vi "Sub Navigation.vi"() -> ()   [LabVIEW 2020]
uses:
  command.ctl
  <vilib>/regexp/Match Regular Expression.xnode
panel:
  out "Answer":i32
  in  "Input":string="forward 1\ndown 6\ndown 6\nforward 2\nforward 2\ndown 2\ndown 1\ndown 5\ndown 7\ndown 3\nforward 1\nforward 6\nup 2\nforward 2\nforward 7\nforward 4\ndown 2\nforward 6\nforward 6\ndown 3\nup 7\ndown 6\nforward 2\nup 5\ndown 7\nforward 8\ndown 8\nforward 8\ndown 5\ndown 5\ndown 8\nforward 9\ndown 7\nforward 9\nforward 9\nforward 8\ndown 6\ndown 9\ndown 1\nforward 8\ndown 6\ndown 7\nup 3\nforward 5\ndown 1\ndown 7\nup 8\nforward 6\ndown 2\ndown 9\ndown 9\nforward 1\ndown 2\ndown 9\nforward 1\nforward 3\ndown 6\nup 7\ndown 7\nforward 3\ndown 4\ndown 3\nup 7\nup 7\nforward 2\ndown 7\nforward 2\ndown 3\nup 7\ndown 7\nforward 6\ndown 2\ndown 7\nforward 5\ndown 9\ndown 2\nup 7\ndown 1\nforward 5\ndown 5\nforward 9\ndown 6\ndown 3\ndown 7\ndown 8\ndown 3\nup 4\ndown 6\nforward 6\nup 7\nup 2\nforward 3\nup 1\ndown 5\nforward 9\nup 3\nforward 8\nup 4\ndown 7\ndown 8\ndown 3\ndown 7\nforward 5\nup 6\ndown 4\ndown 8\ndown 8\nforward 7\ndown 5\nforward 3\nforward 1\ndown 1\nforward 1\nup 1\nforward 4\nforward 9\nup 8\ndown 7\ndown 9\ndown 1\ndown 2\ndown 1\ndown 4\nforward 4\nforward 8\nforward 6\nforward 1\nforward 6\nforward 9\ndown 1\nup 9\ndown 9\nforward 2\ndown 6\ndown 8\ndown 6\nup 7\nforward 2\nup 2\nforward 5\ndown 2\nup 2\nup 9\nforward 7\ndown 6\nforward 3\ndown 5\nup 4\ndown 1\ndown 5\ndown 6\nup 7\ndown 3\ndown 9\nup 8\ndown 2\nup 8\ndown 1\ndown 2\ndown 4\nforward 6\nup 7\nup 3\nforward 8\ndown 9\ndown 8\nforward 3\nup 5\nforward 1\ndown 5\nup 2\ndown 5\nup 4\ndown 6\nforward 9\ndown 1\ndown 1\nforward 1\ndown 2\nforward 9\nup 5\ndown 7\nforward 7\ndown 9\ndown 5\ndown 3\nforward 4\ndown 2\nforward 7\nforward 3\nup 4\ndown 9\nforward 9\nforward 3\nforward 1\nforward 6\ndown 1\ndown 5\ndown 3\nforward 9\ndown 2\nforward 9\nup 7\nforward 7\nforward 7\nforward 8\nforward 6\nforward 5\ndown 7\nup 4\nforward 7\nup 2\nforward 6\ndown 2\ndown 9\ndown 3\nforward 5\ndown 3\ndown 9\nforward 2\nup 4\nforward 7\nforward 3\nforward 8\ndown 4\nforward 4\ndown 3\nup 7\nup 1\nup 4\ndown 3\ndown 5\ndown 3\ndown 7\ndown 3\ndown 7\ndown 5\ndown 1\nforward 5\nforward 6\ndown 1\nforward 9\ndown 4\nup 1\nforward 5\nup 6\ndown 4\nup 7\ndown 4\ndown 9\nforward 7\nup 8\nforward 3\nforward 5\ndown 9\ndown 1\ndown 7\nforward 9\ndown 9\ndown 5\nforward 6\nforward 4\nforward 3\ndown 1\ndown 2\nup 4\nup 7\ndown 8\nforward 4\nforward 1\nforward 8\ndown 8\ndown 8\nforward 1\nforward 5\nup 8\nforward 2\ndown 6\nforward 6\ndown 6\nforward 7\ndown 9\ndown 4\nup 4\nup 5\ndown 7\nforward 4\ndown 7\ndown 5\nforward 7\ndown 3\ndown 2\nforward 5\nforward 1\ndown 5\ndown 4\ndown 8\nup 8\nforward 3\ndown 7\ndown 8\ndown 5\nforward 1\ndown 6\nforward 8\nforward 2\nforward 3\ndown 4\nup 3\ndown 4\nforward 3\nforward 9\nup 5\nup 9\ndown 3\nup 4\nforward 4\ndown 9\nforward 8\ndown 2\ndown 2\nforward 9\ndown 5\ndown 2\nup 1\nforward 6\nforward 4\nup 5\nup 3\nup 8\ndown 7\nforward 5\nup 7\nforward 9\ndown 6\ndown 7\nforward 4\ndown 9\nup 2\nforward 8\ndown 1\nforward 6\nforward 1\nforward 4\ndown 9\ndown 6\nup 1\nforward 1\ndown 5\nup 1\nforward 3\ndown 1\ndown 4\nforward 3\ndown 4\nup 9\ndown 6\nup 6\nforward 1\nforward 8\nup 1\ndown 7\nup 8\nup 3\nup 7\ndown 9\nforward 8\ndown 3\nup 2\nforward 3\nup 4\nup 3\ndown 5\nforward 3\nforward 2\ndown 3\nforward 5\nup 4\ndown 9\ndown 8\ndown 3\ndown 5\ndown 7\nforward 2\nforward 8\nup 9\nforward 9\ndown 4\ndown 8\nforward 5\ndown 2\nup 4\ndown 7\nforward 6\nup 9\nforward 6\ndown 9\ndown 5\nforward 9\ndown 5\ndown 3\nup 6\nup 6\ndown 7\nup 1\nforward 7\nforward 4\ndown 5\nforward 8\ndown 5\ndown 8\nforward 4\nforward 8\nforward 1\ndown 7\nforward 4\ndown 6\ndown 4\nup 8\ndown 4\nup 5\nup 7\nup 2\ndown 5\ndown 9\nforward 6\ndown 7\ndown 9\ndown 3\nup 4\ndown 8\nforward 3\nforward 5\nforward 8\ndown 9\nforward 9\ndown 1\nup 1\ndown 9\nforward 3\nup 9\nforward 5\nforward 2\ndown 1\ndown 5\ndown 6\nforward 5\nforward 4\nup 5\nforward 5\nup 4\nup 9\nup 4\nforward 8\ndown 7\ndown 6\ndown 9\ndown 3\ndown 2\ndown 6\nup 6\nforward 6\nup 3\ndown 3\nforward 3\ndown 2\ndown 9\ndown 3\nforward 1\nforward 8\ndown 2\ndown 9\ndown 6\nup 3\ndown 6\nforward 1\nforward 1\nforward 2\ndown 9\ndown 8\nforward 9\ndown 2\nup 3\nforward 2\nup 5\nup 8\ndown 4\nup 3\nforward 3\nforward 5\nforward 1\ndown 5\nup 4\nforward 4\ndown 7\nforward 8\nup 7\nforward 5\ndown 2\nforward 4\nforward 6\ndown 7\ndown 9\nforward 2\nforward 2\ndown 4\ndown 5\nup 5\nforward 5\nforward 2\ndown 8\nforward 6\ndown 1\ndown 6\nforward 1\ndown 8\nup 6\ndown 8\nforward 4\ndown 4\ndown 4\nforward 3\nup 8\ndown 1\nforward 7\ndown 5\nforward 1\ndown 9\ndown 9\ndown 5\nforward 1\ndown 4\nup 6\nforward 4\nforward 5\nforward 1\ndown 4\ndown 2\ndown 5\nforward 6\nforward 1\nforward 6\ndown 2\ndown 6\nforward 3\ndown 9\nup 6\nforward 2\nup 7\nforward 8\ndown 7\nup 1\nforward 1\ndown 8\nforward 8\ndown 9\nforward 4\ndown 4\ndown 5\ndown 8\nup 3\nforward 1\nforward 9\ndown 9\nup 2\ndown 1\ndown 8\ndown 6\nforward 3\ndown 8\ndown 3\nforward 5\nforward 2\nforward 5\nforward 5\nforward 2\nforward 4\ndown 9\ndown 3\nforward 7\nforward 3\nup 3\nup 1\nforward 2\ndown 5\nforward 3\nup 3\nforward 2\nforward 9\nforward 5\ndown 3\nforward 9\nup 2\nforward 7\nup 3\ndown 8\nforward 7\nup 5\nforward 3\nforward 4\nup 5\ndown 6\nup 2\nforward 8\nup 3\ndown 5\ndown 4\nforward 9\nup 2\ndown 5\nforward 4\nup 7\ndown 9\nup 8\ndown 4\nup 5\nforward 4\ndown 8\nforward 3\ndown 5\ndown 5\ndown 8\nup 9\nforward 3\nforward 9\ndown 2\nforward 4\ndown 1\nup 3\ndown 9\nup 6\ndown 1\ndown 1\ndown 5\ndown 1\ndown 7\nforward 4\ndown 4\ndown 9\nup 1\nup 7\nup 2\ndown 8\nup 5\ndown 6\nforward 6\nforward 6\ndown 4\nforward 9\nforward 4\nforward 9\nforward 4\nup 5\nforward 9\nup 7\nup 1\nforward 5\nforward 9\ndown 7\nforward 7\nforward 6\ndown 5\nforward 9\nup 9\ndown 4\ndown 9\ndown 2\nforward 3\ndown 3\ndown 3\nforward 9\ndown 8\ndown 4\ndown 8\ndown 6\ndown 6\ndown 9\nup 5\ndown 3\ndown 4\nup 6\nup 2\nforward 1\nup 9\nup 9\nforward 9\nforward 7\ndown 3\nforward 2\nup 5\ndown 2\nforward 2\nforward 8\ndown 8\nforward 4\nforward 2\nup 3\nup 8\ndown 5\nforward 5\nforward 8\ndown 1\ndown 8\nforward 3\nforward 9\ndown 7\nforward 5\nforward 8\nforward 1\nup 6\nforward 9\nup 5\nforward 8\nforward 3\ndown 2\nup 9\nup 7\nforward 5\ndown 8\ndown 3\nforward 8\ndown 3\ndown 9\ndown 9\nforward 7\ndown 9\nforward 5\nforward 1\nforward 5\ndown 2\ndown 7\nforward 4\ndown 4\nup 8\ndown 2\nup 1\ndown 1\nup 5\nup 6\ndown 5\nup 9\nup 6\ndown 6\ndown 4\ndown 3\nforward 9\nforward 2\nforward 2\nup 6\nforward 9\ndown 3\nforward 4\nforward 6\nforward 8\nforward 2\nforward 8\nforward 4\ndown 1\nforward 3\nup 1\nup 9\nforward 9\nup 6\nup 5\nforward 2\ndown 6\nup 8\nup 9\nforward 3\nforward 9\ndown 7\ndown 6\nforward 2\ndown 7\nforward 4\ndown 5\ndown 2\ndown 6\ndown 2\ndown 5\ndown 3\nforward 3\ndown 7\ndown 6\ndown 5\nup 2\nforward 4\nup 9\nforward 2\nforward 4\ndown 5\nup 9\nup 2\nforward 9\nforward 6\ndown 6\ndown 3\ndown 5\ndown 1\nup 4\nup 1\ndown 4\ndown 1\nforward 5\nforward 3\ndown 7\ndown 9\nforward 2\ndown 3\nup 7\ndown 2\ndown 6\nforward 3\nforward 3\ndown 3\nup 1\nforward 6\nforward 3\ndown 6\ndown 2\nup 4\nup 3\ndown 5\ndown 9\ndown 3\nforward 7\nforward 2\nforward 9\ndown 6\nforward 4\nup 9\nforward 1\ndown 4\ndown 6\ndown 2\nforward 3\ndown 2\nup 8\nforward 1\nforward 9\ndown 9\nup 7\nforward 6\nup 8\ndown 9\ndown 4\nforward 8\ndown 6\ndown 1\ndown 9\ndown 1\nup 7\nforward 9\nup 3\nforward 7\nup 7\ndown 2\nforward 1\ndown 4\ndown 7\nforward 7\nforward 9\ndown 6\ndown 5\ndown 8\ndown 9\nup 3\ndown 7\nup 3\ndown 1\nforward 1\nforward 6\nforward 2\ndown 6\nforward 9\nforward 1\nup 2\nforward 1\nforward 3\nforward 4\nforward 7\nforward 4\ndown 3\nup 8\nforward 9\ndown 7\nforward 6\nforward 3\ndown 6\nforward 4\nup 1\nforward 3\ndown 3\nforward 9\nforward 2\nforward 1\nforward 4\nup 6\nforward 3\ndown 6\ndown 8\nup 4\nforward 8\nforward 4\ndown 8\nup 4\nup 3\nforward 9\nforward 3\ndown 5\nforward 7\nforward 1\nup 8\nup 4\ndown 1\ndown 3\ndown 9\ndown 7\nup 5\nforward 6\ndown 1\nforward 3\ndown 2\ndown 2\ndown 6\nforward 2\ndown 5\nforward 2\nforward 1\nup 9\ndown 1\nforward 3\ndown 3\nforward 6\ndown 1\nforward 5\nforward 7\ndown 6\nforward 7\ndown 4\nup 7\nforward 1\ndown 7\ndown 8\ndown 9\ndown 6\ndown 1\nforward 6\ndown 7\nforward 2\ndown 2\nup 1\nup 2\ndown 3\ndown 4\nup 2\nforward 3\ndown 5\ndown 4\ndown 9\ndown 6\ndown 9\ndown 7\ndown 2\nforward 7\nforward 3\nup 3\ndown 1\ndown 5\ndown 1\ndown 3\ndown 3\nforward 9\ndown 1\ndown 7\nup 4\ndown 1\ndown 6\nup 9\ndown 9\nforward 6\ndown 9\nforward 3\nforward 8\nup 1\nforward 3\ndown 8\nforward 2\ndown 6\ndown 1\nup 7\ndown 1\nforward 3\ndown 2\nforward 1\nup 8\nforward 8\nforward 7\ndown 9\nforward 3"
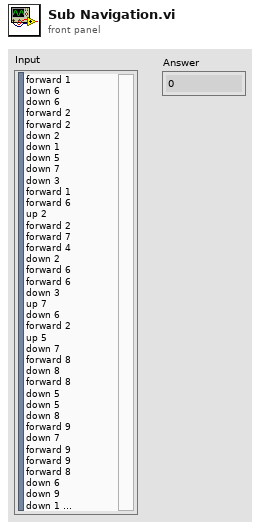
[diagram p1: front panel]
types:
  T1 = typedef "command.ctl" = enum16{"forward", "down", "up"}
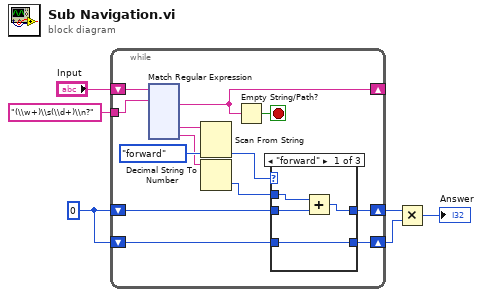
[diagram p0: block diagram]
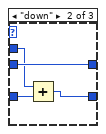
[diagram p2: hidden frame]
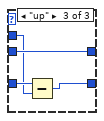
[diagram p3: hidden frame]
diagram:
  w4 = 0
  n1 = while {
    shift-right: [w17] -> _
    shift-left: "Input" -> [w19]
    tunnel: "(\\w+)\\s(\\d+)\\n?" -> [w18]
    shift-right: [w7] -> w3
    shift-left: w4 -> [w10]
    shift-right: [w8] -> w2
    shift-left: w4 -> [w9]
    stop <- w16 stop-if-true
    n2 = xnode "Match Regular Expression"("input string"=w19, "regular expression"=w18) -> ("after match"=w17:string, "submatch 1"=w15:string, "submatch 2"=w13:string)  [unwired: 4 in, 4 out]
    n3 = Scan From String(input string=w15, default 1=command."forward" ("command")) -> (output 1=w12:T1)  [unwired: 3 in, 3 out]
    n4 = Decimal String To Number(string=w13) -> (number=w11:i32)  [unwired: 2 in, 1 out]
    n5 = Empty String/Path?(string/path=w17) -> (empty?=w16:bool)
    n6 = case shown="\"forward\"" w12 {
      tunnel: w11 -> [w22 w25 w29]
      tunnel: w10 -> [w23 w27 w31]
      tunnel: w9 -> [w21 w26 w30]
      tunnel: [w21 w24 w28] -> w8
      tunnel: [w20 w27 w31] -> w7
      frame "forward" {
        n7 = Add(x=w22, y=w23) -> (x+y=w20:i32)
      }
      frame "down" {
        n8 = Add(x=w25, y=w26) -> (x+y=w24:i32)
      }
      frame "up" {
        n9 = Subtract(x=w30, y=w29) -> (x-y=w28:i32)
      }
    }
  }
  n10 = Multiply(x=w3, y=w2) -> (x*y=→"Answer":i32)
